vi "CheckFinish.vi"(0 "object in":refnum<class "PassPlay_v2.lvclass">, 3 "GameRef":refnum<data-value>, 5 "error in (no error)":errorcluster) -> (14 "object out":refnum<class "PassPlay_v2.lvclass">, 16 "finish":bool, 18 "playIndex":u8, 19 "error out":errorcluster)   [LabVIEW 2023, in "PassPlay_v2.lvclass"]
uses:
  PassPlay_v2.lvclass
  Game_class/Game.lvclass
  Play_v2_class/Play_v2.lvclass
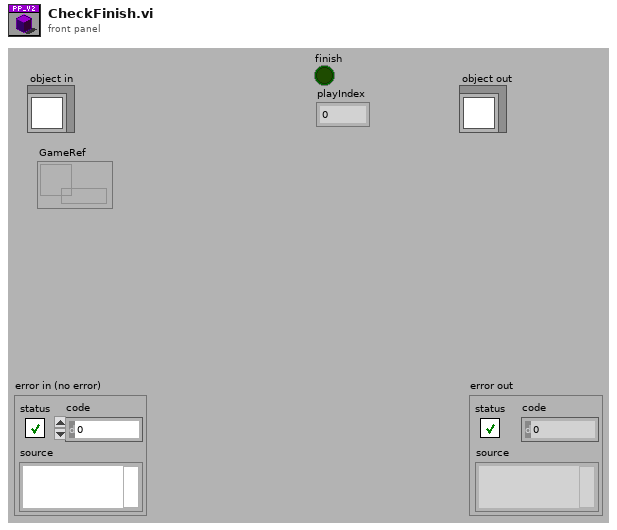
[diagram p1: front panel]
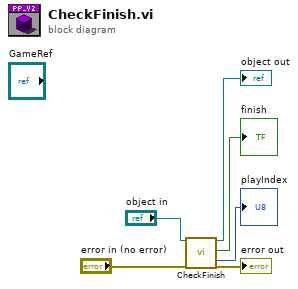
[diagram p0: block diagram]
diagram:
  n1 = call-parent "CheckFinish.vi"("object in"="object in", "error in (no error)"="error in (no error)") -> ("object out"=→"object out":refnum<class "PassPlay_v2.lvclass">, "finish"=→"finish":bool, "playIndex"=→"playIndex":u8, "error out"=→"error out":errorcluster)  [unwired: 14 in]
